vi "JSON Pop.vi"(6 "Pretty Print? (F)":bool, 8 "error in (no error)":errorcluster, 9 "Default":variant, 10 "Root Path ([]=Root)":string[](array[string]), 11 "JSON in":string) -> (0 "error out":errorcluster, 1 "Value":variant, 2 "Exists?":bool, 3 "JSON out":string)   [LabVIEW 2019, in "labview_json.lvlib"]
doc: "Pop an element from the <b>JSON in</b> string. \nIf the element is not found, <b>Default</b> is returned. \nSpecify the <b>Root Path</b> to the nested object key or array index. \nIf <b>Default</b> is not specified, this returns the native JSON types. \n<b>Exists?</b> only returns True if all elements are found.\n<b>Pretty Print?</b> whitespace indents the <b>JSON out</b> string.\nCreated by: Ryan Pacini"
uses:
  labview_json.lvlib
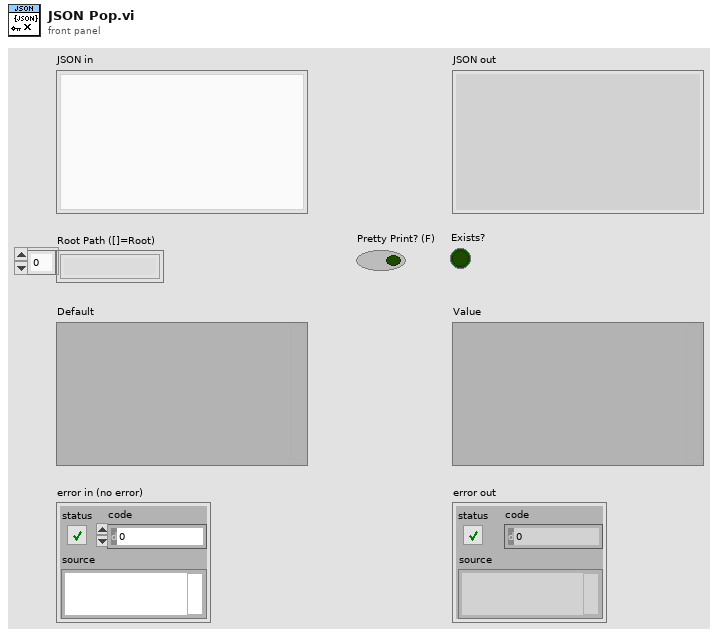
[diagram p1: front panel]
types:
  T1 = typedef "labview_json.lvlib/Element.ctl" = cluster{"Key":string, "Type":T2, "Value":variant, "IsRootPath":bool}
  T2 = typedef "labview_json.lvlib/Element Type.ctl" = enum8{"NULL", "OBJECT", "ARRAY", "BOOL", "INT", "UINT", "FLOAT", "STRING"}
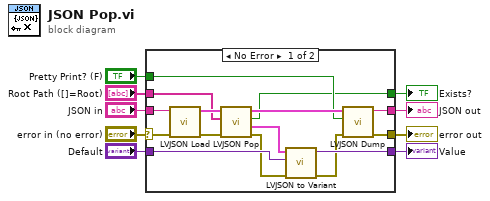
[diagram p0: block diagram]
diagram:
  n1 = case shown="No Error" "error in (no error)" {
    selector: "error in (no error)" -> [w24 w27]
    tunnel: [w23 w27] -> w8
    tunnel: "JSON in" -> [w22 w26]
    tunnel: [w21 w26] -> w6
    tunnel: "Root Path ([]=Root)" -> [w18 _]
    tunnel: "Default" -> [w16 w25]
    tunnel: [w15 w25] -> w3
    tunnel: "Pretty Print? (F)" -> [w12 _]
    tunnel: [w11 _] -> w1
    frame No Error {
      n2 = call "LVJSON Load.vi"("error in (no error)"=w24, "JSON in"=w22) -> ("error out"=w10:errorcluster, "Root Element out"=w20:T1)  [unwired: 8 in]
      n3 = call "LVJSON Pop.vi"("error in (no error)"=w10, "Root Path"=w18, "Root Element in"=w20) -> ("error out"=w14:errorcluster, "Element out"=w17:T1, "Exists?"=w11:bool, "Root Element out"=w19:T1)  [unwired: 5 in]
      n4 = call "LVJSON to Variant.vi"("error in (no error)"=w14, "Variant Type"=w16, "Root Element in"=w17) -> ("error out"=w13:errorcluster, "Variant out"=w15:variant)  [unwired: 6 in, 1 out]
      n5 = call "LVJSON Dump.vi"("error in (no error)"=w13, "Pretty Print? (F)"=w12, "Root Element in"=w19) -> ("error out"=w23:errorcluster, "JSON out"=w21:string)  [unwired: 6 in, 1 out]
    }
    frame Error {
    }
  }
  "error out" <- w8
  "JSON out" <- w6
  "Value" <- w3
  "Exists?" <- w1
